vi "CouchDB2LabView.vi"() -> (0 "value":dbl)   [LabVIEW 2011]
doc: "This example demonstrates how to use an event structure to post a message and pass data to the event structure using the PostLVUserEvent() function. The VI calls the dll using the Call Library Function Node, and the dll passes three messages to the event structure. A dialog window displays the data and remains open for 2 seconds. The dll is called in its own thread so it does not hang the UI thread."
uses:
  libs/AccCouchDB.dll
panel:
  out "Abort":i32
  in  "Stop":bool
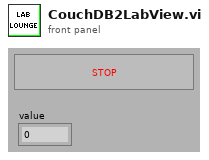
[diagram p1: front panel]
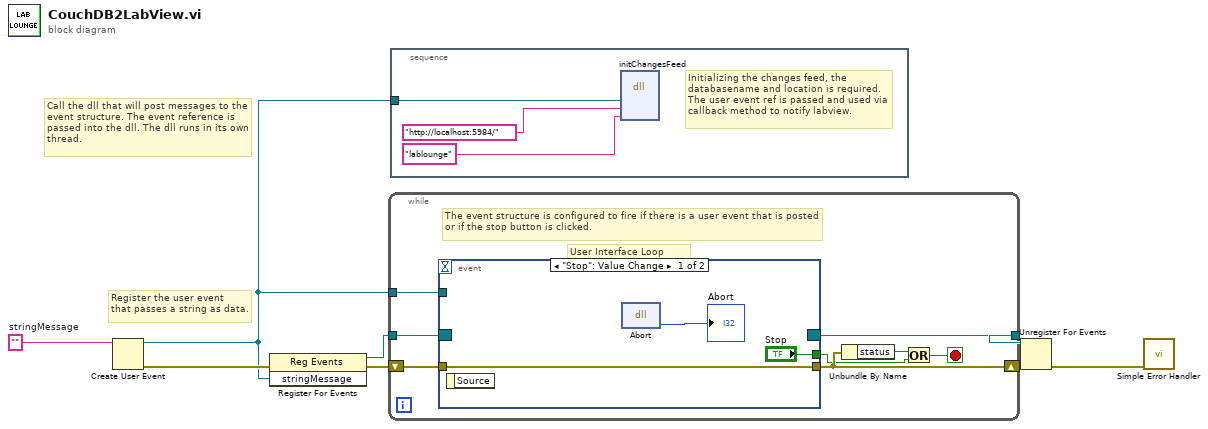
[diagram p0: block diagram]
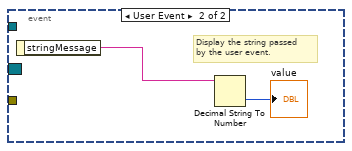
[diagram p2: hidden frame]
diagram:
  w2 = ""  # stringMessage
  # "Initializing the changes feed, the databasename and location is required. The user event ref is passed and used via callback method to notify labview."
  # "Call the dll that will post messages to the event structure. The event reference is passed into the dll. The dll runs in its own thread."
  # "Register the user event \nthat passes a string as data."
  n1 = Create User Event(user event datatype=w2) -> (user event=w1:refnum<user-event>, error out=w3:errorcluster)  [unwired: 1 in]
  n2 = register-events(error in=w3, w1) -> (reference out=w6:refnum<event-registration>, error out=w4:errorcluster)  [unwired: 1 in]
  n3 = while {
    tunnel: w6 -> [w16]
    shift-right: [w14] -> w7
    shift-left: w4 -> [w15]
    tunnel: [w13] -> w5
    tunnel: w1 -> [w9]
    stop <- w11 stop-if-true
    # "The event structure is configured to fire if there is a user event that is posted or if the stop button is clicked."
    # "User Interface Loop"
    n4 = event shown="[0] \"Stop\": Value Change" {
      selector: w16 -> [_ _]
      dyn-events: [_ _] -> w13
      timeout: _ -> [_ _]
      tunnel: ["Stop" _] -> w10
      tunnel: w15 -> [w18 _]
      tunnel: [w18 _] -> w14
      tunnel: w9 -> [_ _]
      event "Stop": Value Change {
        n5 = event-data() -> ()  [unwired: 1 in, 1 out]
        n6 = dll-call lib="C:/projects/libs/AccCouchDB.dll" fn="Abort"() -> ("return type"=→"Abort":i32)  [unwired: 3 in, 2 out]
      }
      event User Event {
        # "Display the string passed\nby the user event."
        n7 = event-data() -> ("stringMessage"=w21:string)  [unwired: 1 in]
        n8 = Decimal String To Number(string=w21) -> (number=→"value":i32)  [unwired: 2 in, 1 out]
      }
    }
    n9 = Unbundle By Name(w14) -> ("status"=w12:bool)
    n10 = Or(x=w12, y=w10) -> (x .or. y?=w11:bool)
  }
  n11 = stacked-sequence {
    tunnel: w1 -> [w24]
    frame #0 {
      n12 = dll-call lib="C:/projects/libs/AccCouchDB.dll" fn="initChangesFeed"("UserEventRef"=w24, "server"="http://localhost:5984/", "database"="lablounge") -> ()  [unwired: 7 in, 2 out]
    }
  }
  n13 = Unregister For Events(event registration refnum=w5, error in=w7) -> (error out=w8:errorcluster)
  n14 = call <vilib>:"Simple Error Handler.vi"("error in (no error)"=w8) -> ()  [unwired: 4 in, 5 out]
